vi "Image_Bidirectional_Inversion.vi"(8 "error in":errorcluster, 11 "Original image":dbl[][](graph)=array100x100[10000 elements]) -> (0 "error out":errorcluster, 3 "Bidirectional corrected image":dbl[][](graph))   [LabVIEW 2025]
doc: "VI qui intervertit une ligne sur deux.\nPermet de réassigner correctement des pixels lors d'un scan bi-directionnel.\n\n->\n<-\n\ndevient\n\n->\n->"
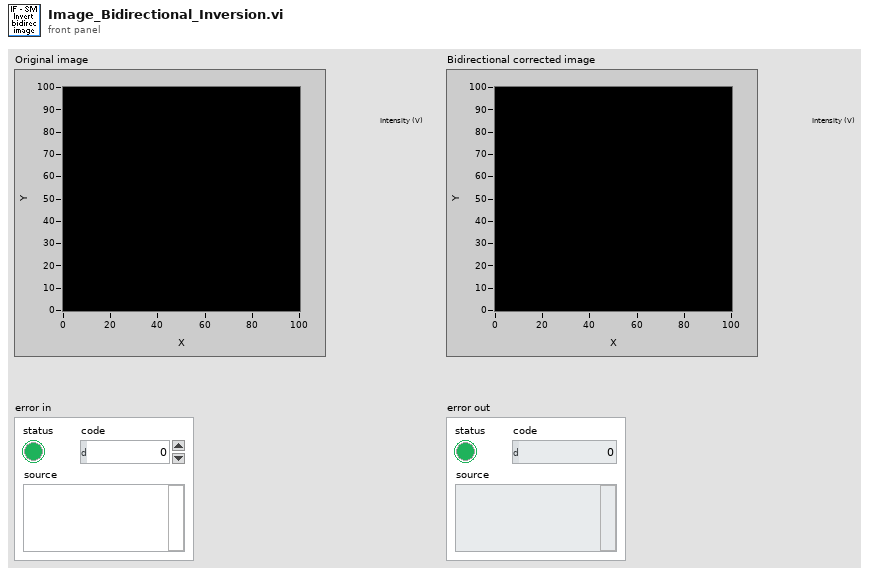
[diagram p1: front panel]
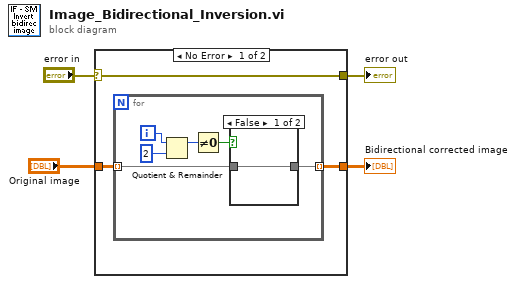
[diagram p0: block diagram]
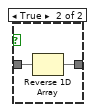
[diagram p2: hidden frame]
diagram:
  n1 = case shown="No Error" "error in" {
    selector: "error in" -> [w7 w18]
    tunnel: [w7 w18] -> w3
    tunnel: "Original image" -> [w6 w17]
    tunnel: [w5 w17] -> w1
    frame No Error {
      n2 = for {
        tunnel: w6 -> [w9] mode=indexing
        tunnel: [w8] -> w5 mode=indexing
        i -> [w10]
        n3 = Quotient & Remainder(x=w10, y=2) -> (x-y*floor(x/y)=w12:i32)  [unwired: 1 out]
        n4 = Not Equal To 0?(x=w12) -> (x != 0?=w11:bool)
        n5 = case shown="False" w11 {
          tunnel: [w14 w15] -> w8
          tunnel: w9 -> [w14 w16]
          frame False {
          }
          frame True {
            n6 = Reverse 1D Array(array=w16) -> (reversed array=w15:dbl[])
          }
        }
      }
    }
    frame Error {
    }
  }
  "error out" <- w3
  "Bidirectional corrected image" <- w1
